vi "Register Diagram Hierarchy in Selection.vi"(8 "error in":errorcluster, 10 "Diag Ref":refnum<vi>, 11 "Selection in":T1) -> (0 "error out":errorcluster, 3 "Selection out":T1)   [LabVIEW 2020, in "Enclose in Structure.lvlib"]
uses:
  Enclose in Structure.lvlib
  <vilib>/Utility/miscctls.llb/LVMapReplaceAction.ctl
  Selection Map.ctl
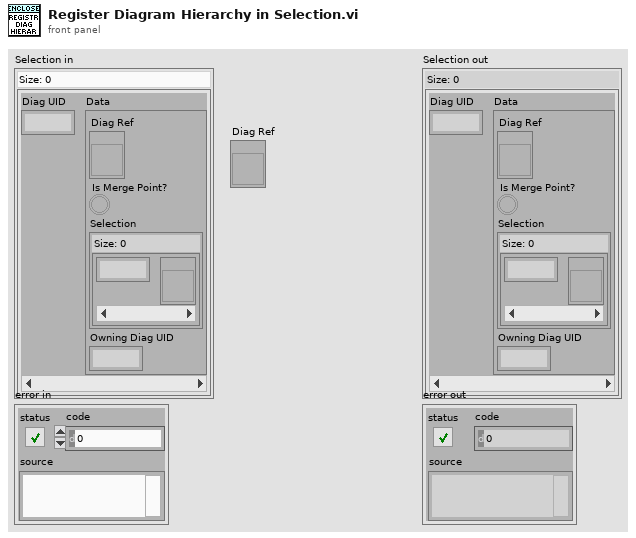
[diagram p1: front panel]
types:
  T1 = typedef "Enclose in Structure.lvlib/Selection Map.ctl" = map{i32, cluster{"Diag Ref":refnum<vi>, "Is Merge Point?":bool, "Selection":map{i32, refnum<vi>}, "Owning Diag UID":i32}}
  T2 = typedef "LVMapReplaceAction.ctl" = enum32{"Modify Entry only if found", "Add or Modify Entry", "Delete Entry"}
  T3 = cluster{"Diag Ref":refnum<vi>, "Is Merge Point?":bool, "Selection":map{i32, refnum<vi>}, "Owning Diag UID":i32}
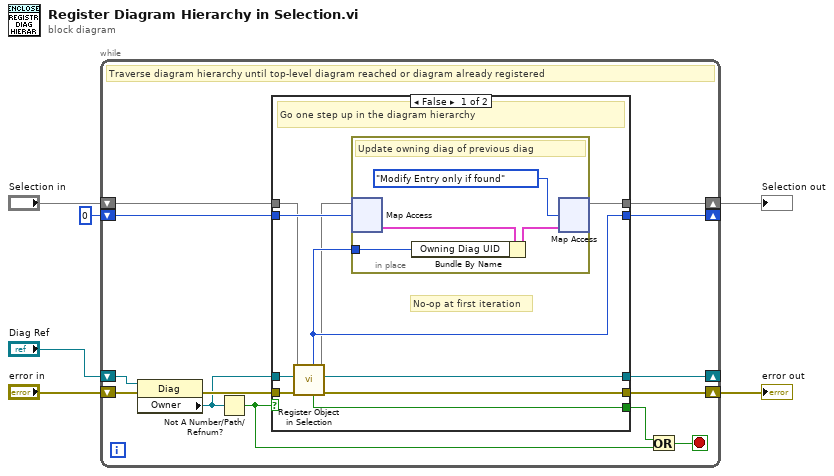
[diagram p0: block diagram]
diagram:
  n1 = while {
    shift-right: [w13] -> w6
    shift-left: "error in" -> [w19]
    shift-right: [w12] -> _
    shift-left: "Diag Ref" -> [w17]
    shift-right: [w14] -> w1
    shift-left: "Selection in" -> [w15]
    shift-right: [w8] -> _
    shift-left: 0 ("Owning Diag UID") -> [w7]
    stop <- w10 stop-if-true
    # "Traverse diagram hierarchy until top-level diagram reached or diagram already registered"
    n2 = property class="Diag"(reference=w17, error in=w19) -> (error out=w18:errorcluster, "Owner"=w16:refnum<vi>)  [unwired: 1 out]
    n3 = Not A Number/Path/Refnum?(number/path/refnum=w16) -> (NaN/Path/Refnum?=w11:bool)
    n4 = case shown="False" w11 {
      tunnel: w18 -> [w28 w35]
      tunnel: [w24 _] -> w12
      tunnel: w16 -> [w27 _]
      tunnel: w15 -> [w21 w34]
      tunnel: [w23 w34] -> w14
      tunnel: [w26 w35] -> w13
      tunnel: [w25 _] -> w9
      tunnel: [w22 _] -> w8
      tunnel: w7 -> [w29 _]
      frame False {
        # "No-op at first iteration"
        # "Go one step up in the diagram hierarchy"
        n5 = call "Register Object in Selection.vi"("error in"=w28, "Object"=w27, "Selection in"=w21) -> ("error out"=w26:errorcluster, "Owning Diag Ref"=w24:refnum<vi>, "Selection out"=w20:T1, "Owning Diag Already Registered?"=w25:bool, "Owning Diag UID"=w22:i32)  [unwired: 4 in]
        n6 = in-place {
          in-place-border: w22 -> [w31]
          # "Update owning diag of previous diag"
          n7 = in-place-map #1(w20, w29) -> (w33:T3)  [unwired: 1 in, 1 out]
          n8 = Bundle By Name(cluster=w33, "Owning Diag UID"=w31) -> (w32:T3)
          n9 = in-place-map #1(w32, LVMapReplaceAction."Modify Entry only if found" ("action")) -> (w23:T1)  [unwired: 2 out]
        }
      }
      frame True {
        # "Top-level diagram reached"
      }
    }
    n10 = Or(x=w9, y=w11) -> (x .or. y?=w10:bool)
  }
  "error out" <- w6
  "Selection out" <- w1
